vi "Export Table.vi"(8 "error in (no error)":errorcluster, 9 "Data":string[][](array[string]), 10 "Column Header Strings[]":string[](array[string]), 11 "MYSQL Database in":refnum<class "MYSQL Database.lvclass">) -> (0 "error out":errorcluster, 3 "MYSQL Database out":refnum<class "MYSQL Database.lvclass">)   [LabVIEW 2023, in "HardwareAbstractionLayer_LVOOP.lvlib" / "MYSQL Database.lvclass"]
uses:
  MYSQL Database.lvclass
  <vilib>/Utility/file.llb/Write Delimited Spreadsheet (string).vi
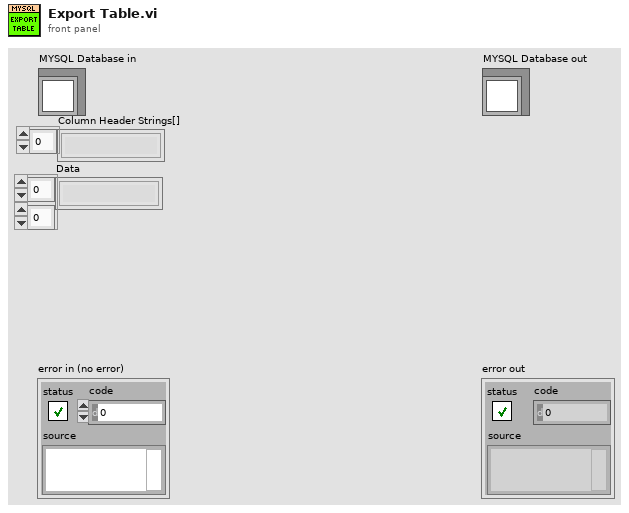
[diagram p1: front panel]
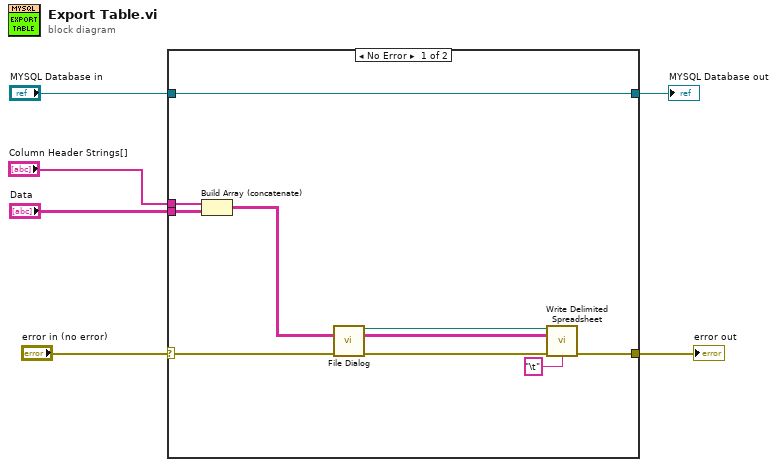
[diagram p0: block diagram]
diagram:
  n1 = case shown="No Error" "error in (no error)" {
    selector: "error in (no error)" -> [w8 w17]
    tunnel: "Column Header Strings[]" -> [w12 _]
    tunnel: "Data" -> [w11 _]
    tunnel: [w7 w17] -> w3
    tunnel: "MYSQL Database in" -> [w9 w16]
    tunnel: [w9 w16] -> w1
    frame No Error {
      n2 = Build Array (concatenate)(w12, w11) -> (w10:string[][])
      n3 = call "File Dialog"("error in"=w8) -> ("selected path"=w14:path, "error out"=w13:errorcluster)  [unwired: 11 in, 2 out]
      n4 = call-poly <vilib>:"Write Delimited Spreadsheet.vi"("file path (dialog if empty)"=w14, "2D data"=w10, "error in (no error)"=w13, "delimiter (\\t)"="\t" ("delimiter (\\t)")) -> ("error out"=w7:errorcluster)  [unwired: 10 in, 1 out]
    }
    frame Error {
    }
  }
  "error out" <- w3
  "MYSQL Database out" <- w1
